vi "re_Tag.write_lua.vi"(5 "LuaVIEW reference":T1) -> (15 "error out":errorcluster)   [LabVIEW 2012]
doc: "Write a point with the given value and an optional timestamp. If the tag has bounds (max and/or min) the value will be clipped to that range. Next the (potentially clipped) value is compared to any limits that are set for the tag. When limits are exceeded, the corresponding handlers are triggered. Exceeded limits do not cause this function to return with an error or prevent the point from being written to the tag.\n\nWhen no timestamp is specified, the time in seconds since the LabVIEW epoch (1-Jan-1904) as obtained via the \"Library Time.vi\" is used. This VI exists to allow custom time sources. Its default implementation simply calls \"Get Date/Time In Seconds\" LabVIEW node, which in turn obtains its time from the system clock. Beware that the system clock has a platform dependent resolution and will drift unless corrected for, e.g. using the ntp protocol.\n\nExplicitly specifying the timestamp might be required when the timing of the values needs a delay correction or is derived from some other source. For example, when the value is derived from other tags, the most recent timestamp of the points used to calculate the value can be copied. When the value is associated with an instrument that uses hardware timing and buffering, the timestamps are best derived from a mutual synchronisation of that hardware clock and the system time.\n\nTimestamps of subsequent points may not decrease and should reflect the time of events in the experimental setup when the value is associated with a sensor or physical setpoint. In practical terms this implies that the timing of sensor values should be lowered by the delay introduced by the sensor-filtering-buffering-driver path, if appreciable. Similarly, the timing of a setpoint should be incremented with the delay introduced by the driver-buffering-filtering-actuator path, if appreciable. \nParameters:\nobj:tag\nnum:value, value of the point to write.\n[num:time], optional timestamp, when omitted the current time is used.\nErrors:\nDead or invalid tag object.\nData logger not initialized."
uses:
  luaview/typedefs/t_LuaVIEW Reference.ctl
  luaview/subvis/private/LuaVIEW Pull (number).vi
  luaview/subvis/private/LuaVIEW Pull (object).vi
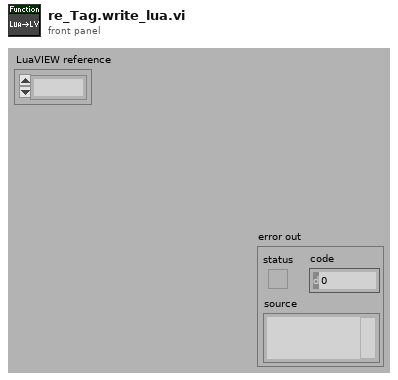
[diagram p1: front panel]
types:
  T1 = typedef "t_LuaVIEW Reference.ctl" = refnum<k1>
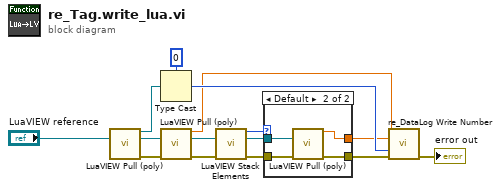
[diagram p0: block diagram]
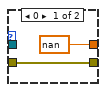
[diagram p2: hidden frame]
diagram:
  n1 = call-poly "LuaVIEW Pull (poly).vi"("LuaVIEW reference in"="LuaVIEW reference") -> ("object refnum"=w13:refnum<vi>, "LuaVIEW reference out"=w9:T1, "error out"=w11:errorcluster)  [unwired: 11 in, 1 out]
  n2 = Type Cast(type=0 ("read index in"), x=w13) -> (*(type *) &x=w10:i32)
  n3 = call-poly "LuaVIEW Pull (poly).vi"("LuaVIEW reference in"=w9, "error in (no error)"=w11) -> ("number"=w2:dbl, "LuaVIEW reference out"=w6:T1, "error out"=w7:errorcluster)  [unwired: 11 in]
  n4 = call "LuaVIEW Stack Elements.vi"("LuaVIEW reference in"=w6, "error in (no error)"=w7) -> ("elements"=w5:i32, "LuaVIEW reference out"=w4:T1, "error out"=w3:errorcluster)  [unwired: 11 in]
  n5 = case shown="Default" w5 {
    tunnel: [w17 w21] -> w15
    tunnel: [nan ("number") w20] -> w1
    tunnel: w4 -> [_ w19]
    tunnel: w3 -> [w17 w18]
    frame 0 {
    }
    frame Default {
      n6 = call-poly "LuaVIEW Pull (poly).vi"("LuaVIEW reference in"=w19, "error in (no error)"=w18) -> ("number"=w20:dbl, "error out"=w21:errorcluster)  [unwired: 11 in, 1 out]
    }
  }
  n7 = call "re_DataLog Write Number.vi"("number"=w2, "time (current)"=w1, "tag index in (use tag)"=w10, "error in (no error)"=w15) -> ("error out"=→"error out":errorcluster)  [unwired: 10 in, 1 out]
